vi "countFilesFromSection.vi"(10 "sectionToCountFiles":string, 11 "text":string) -> (2 "count":u32)   [LabVIEW 2023, in "gitTools.lvlib"]
uses:
  gitTools.lvlib
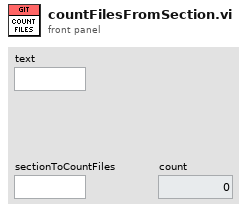
[diagram p1: front panel]
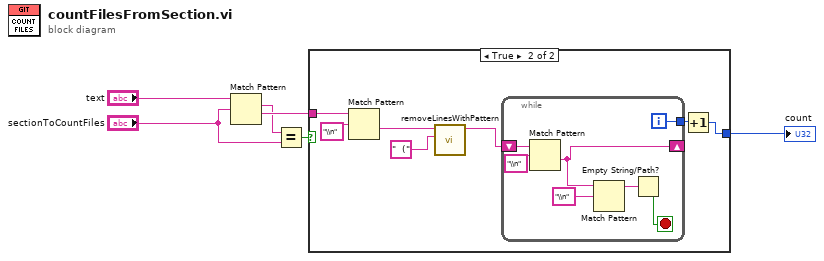
[diagram p0: block diagram]
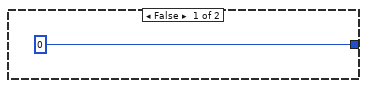
[diagram p2: hidden frame]
diagram:
  n1 = Match Pattern(string="text", regular expression="sectionToCountFiles") -> (match substring=w1:string, after substring=w4:string)  [unwired: 1 in, 2 out]
  n2 = Equal?(x=w1, y="sectionToCountFiles") -> (x = y?=w3:bool)
  n3 = case shown="True" w3 {
    tunnel: w4 -> [_ w14]
    tunnel: [u32 0 w11] -> w5
    frame False {
    }
    frame True {
      n4 = Match Pattern(string=w14, regular expression="\\n") -> (after substring=w10:string)  [unwired: 1 in, 3 out]
      n5 = call "removeLinesWithPattern.vi"("pattern"="  (" ("y"), "text"=w10) -> ("result"=w9:string)  [unwired: 9 in]
      n6 = while {
        tunnel: [w21] -> w12
        shift-right: [w15] -> _
        shift-left: w9 -> [w20]
        i -> [w21]
        stop <- w16 stop-if-true
        n7 = Match Pattern(string=w20, regular expression="\\n") -> (after substring=w15:string)  [unwired: 1 in, 3 out]
        n8 = Match Pattern(string=w15, regular expression="\\n") -> (before substring=w17:string)  [unwired: 1 in, 3 out]
        n9 = Empty String/Path?(string/path=w17) -> (empty?=w16:bool)
      }
      n10 = Increment(x=w12) -> (x+1=w11:i32)
    }
  }
  "count" <- w5
